vi "main.vi"() -> ()   [LabVIEW 2009]
uses:
  subvi/activity_info.vi
  <vilib>/Utility/file.llb/Write To Spreadsheet File (DBL).vi
  <vilib>/Utility/sysdir.llb/System Directory Type.ctl
panel:
  out "Primary and secondary axis power":dbl[](array[slide]) scale=0.0..800.0
  in  "Save Reference Signal to file":bool
  in  "Analysis Interval (s)":dbl(slide)=1.0 scale=0.0..4.0
  in  "Do ANN analysis":bool
  in  "Analysis Upperbound (minutes)":dbl(slide)=1000.0 scale=0.0..30.0
  out "minutes left":dbl
  out "minutes of execution":dbl
  out "case 3":i32
  out "case 2":i32
  out "case 1":i32
  out "case 0":i32
  out "output 2":dbl[](array[slide]) scale=0.0..1.0
  out "Correlations":cluster{dbl[], "correlation array":dbl[]}(graph)
  in  "Slide":cluster{dbl, dbl}(slide)={0.0, 1.0} scale=0.0..1.0
  out "above threshold":dbl(slide) scale=0.0..1.0
  in  "Threshold":dbl(slide)=0.85 scale=0.0..1.0
  out "Analyzing":u8(slide) scale=0.0..100.0
  in  "analyze correlations":bool
  in  "Reference Signal":i32
  in  "Reference Signals":dbl[][](array[numeric])
  in  "Save as reference Signal":bool
  in  "read weights":bool
  in  "Path":path=path "E:/Sensor/data/Phase II Data/csv format/Ara/Ara Walking.csv"
  out "C":bool
  out "B":bool
  out "A":bool
  in  "write data":bool
  out "Fundamental frequency":dbl(slide) scale=0.0..6.0
  in  "Normalize":bool
  in  "write to memory":bool
  out "activity output":u16(ring) items=["A", "B", "C", "D"]
  out "output":dbl[](array[slide]) scale=0.0..1.0
  in  "stop learning":bool
  out "Error (training)":dbl(graph)
  in  "Learning Rate":dbl(slide)=0.336734693877551 scale=0.0..1.0
  in  "Beta":dbl(slide)=1.0 scale=0.0..1.0
  in  "train":bool
  in  "Number of hidden neurons":i32(slide)=9 scale=0.0..20.0
  in  "delete state":bool
  in  "state":u32
  in  "activity":u16(ring) items=["A", "B", "C", "D", "E", "F", "G", "H"]
  in  "save state":bool
  in  "Tab Control":T1(tab)=enum."FFT on data 1"
  out "Time data on X',Y',Z'":T2(graph)
  out "FFT on X',Y',Z'":T3(graph)
  out "Filtered signal":dbl[](graph)
  out "Magnitude of time data":cluster{dbl[], dbl[]}(graph)
  out "activity states":T4(graph)
  in  "Sensor":u16(ring)=1 items=["Sensor 1", "Sensor 2", "Sensor 3"]
  in  "Sensor Type":u16(ring) items=["Acceleration", "Rotation"]
  in  "Sensor Brand":u16(ring)=1 items=["ADXL", "Kinetisense"]
  in  "End time (s) 1":dbl(slide)=10.0 scale=0.0..600.0
  in  "FFT interval (s) 1":dbl(slide)=4.0 scale=0.0..40.0
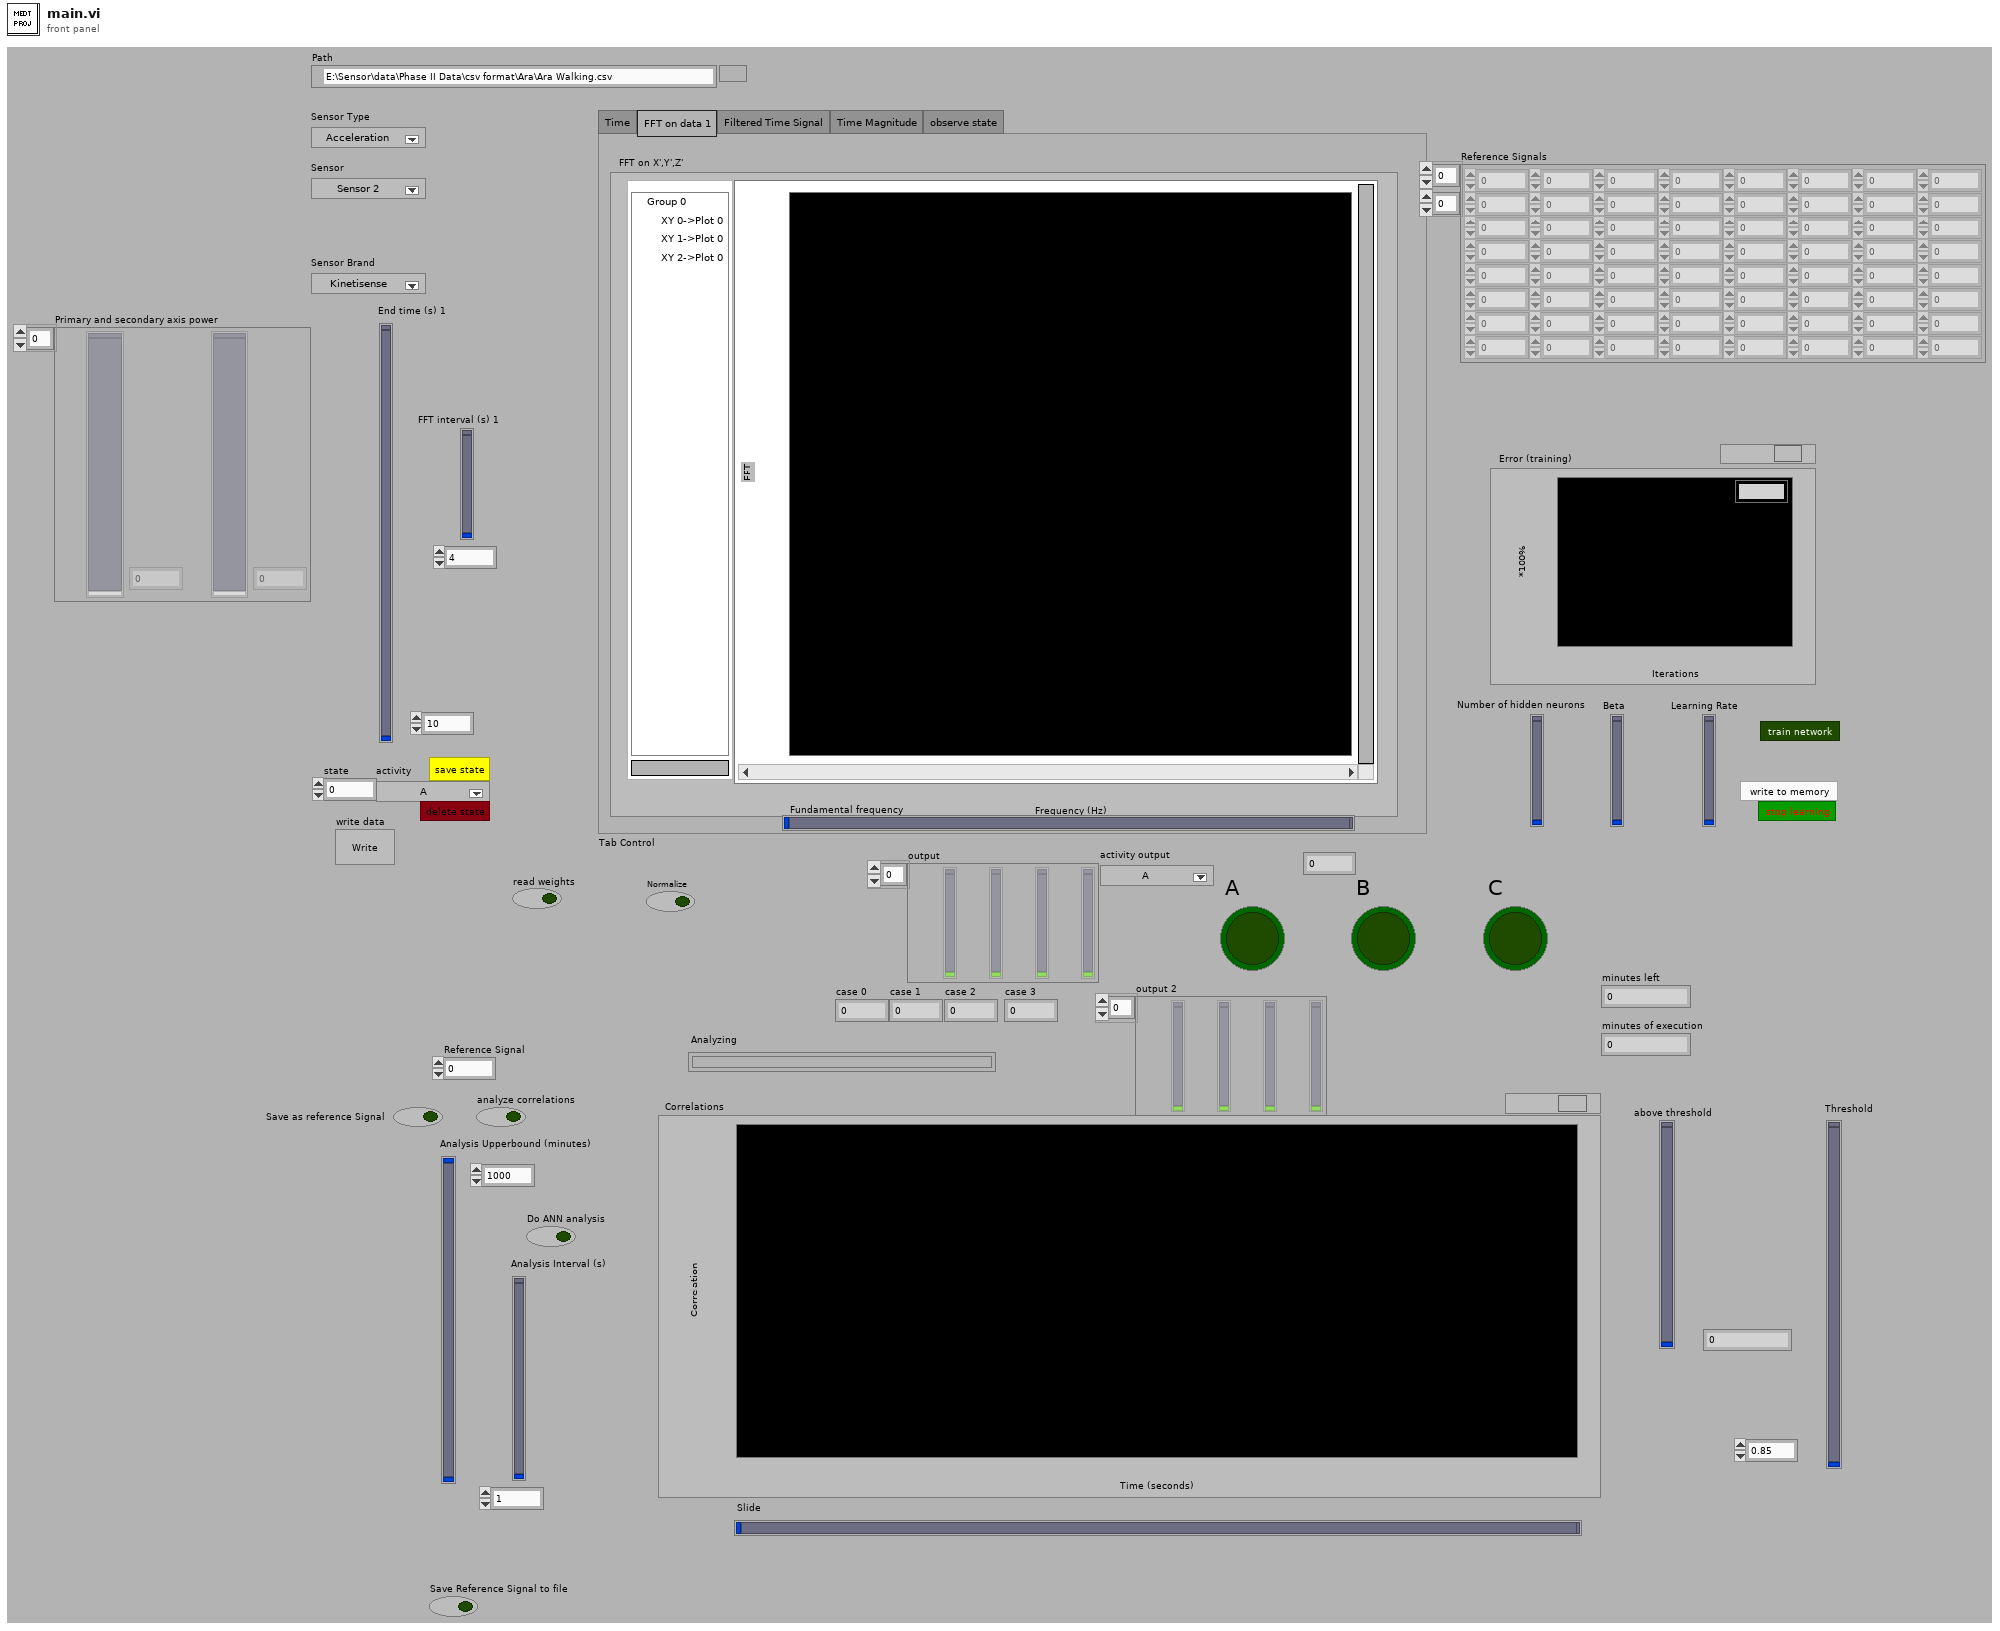
[diagram p1: front panel]
types:
  T1 = enum32{"Time", "FFT on data 1", "Filtered Time Signal", "Time Magnitude", "observe state"}
  T2 = cluster{cluster{dbl[], "Data out":dbl[]}, cluster{dbl[], "Data out":dbl[]}, cluster{dbl[], "Data out":dbl[]}}
  T3 = cluster{"XY Graph":cluster{dbl[], "magnitude":dbl[]}, "XY Graph":cluster{dbl[], "magnitude":dbl[]}, "XY Graph":cluster{dbl[], "magnitude":dbl[]}}
  T4 = cluster{cluster{dbl[], "Bicycling":dbl[]}, cluster{dbl[], "Bicycling":dbl[]}, cluster{dbl[], dbl[]}, cluster{dbl[], dbl[]}, cluster{dbl[], dbl[]}}
  T5 = typedef "System Directory Type.ctl" = i32
  T6 = cluster{"correlation array":dbl[], "correlation array":dbl[]}
  T7 = cluster{"A":dbl[][], "B":dbl[][], "C":dbl[][], "D":dbl[][]}
  T8 = cluster{cluster{dbl[], dbl[]}, cluster{dbl[], dbl[]}, cluster{dbl[], dbl[]}}
  T9 = cluster{"Cluster":cluster{dbl[], "activity":dbl[]}, "Cluster":cluster{dbl[], "activity":dbl[]}, cluster{dbl[], dbl[]}, cluster{dbl[], dbl[]}, cluster{dbl[], dbl[]}}
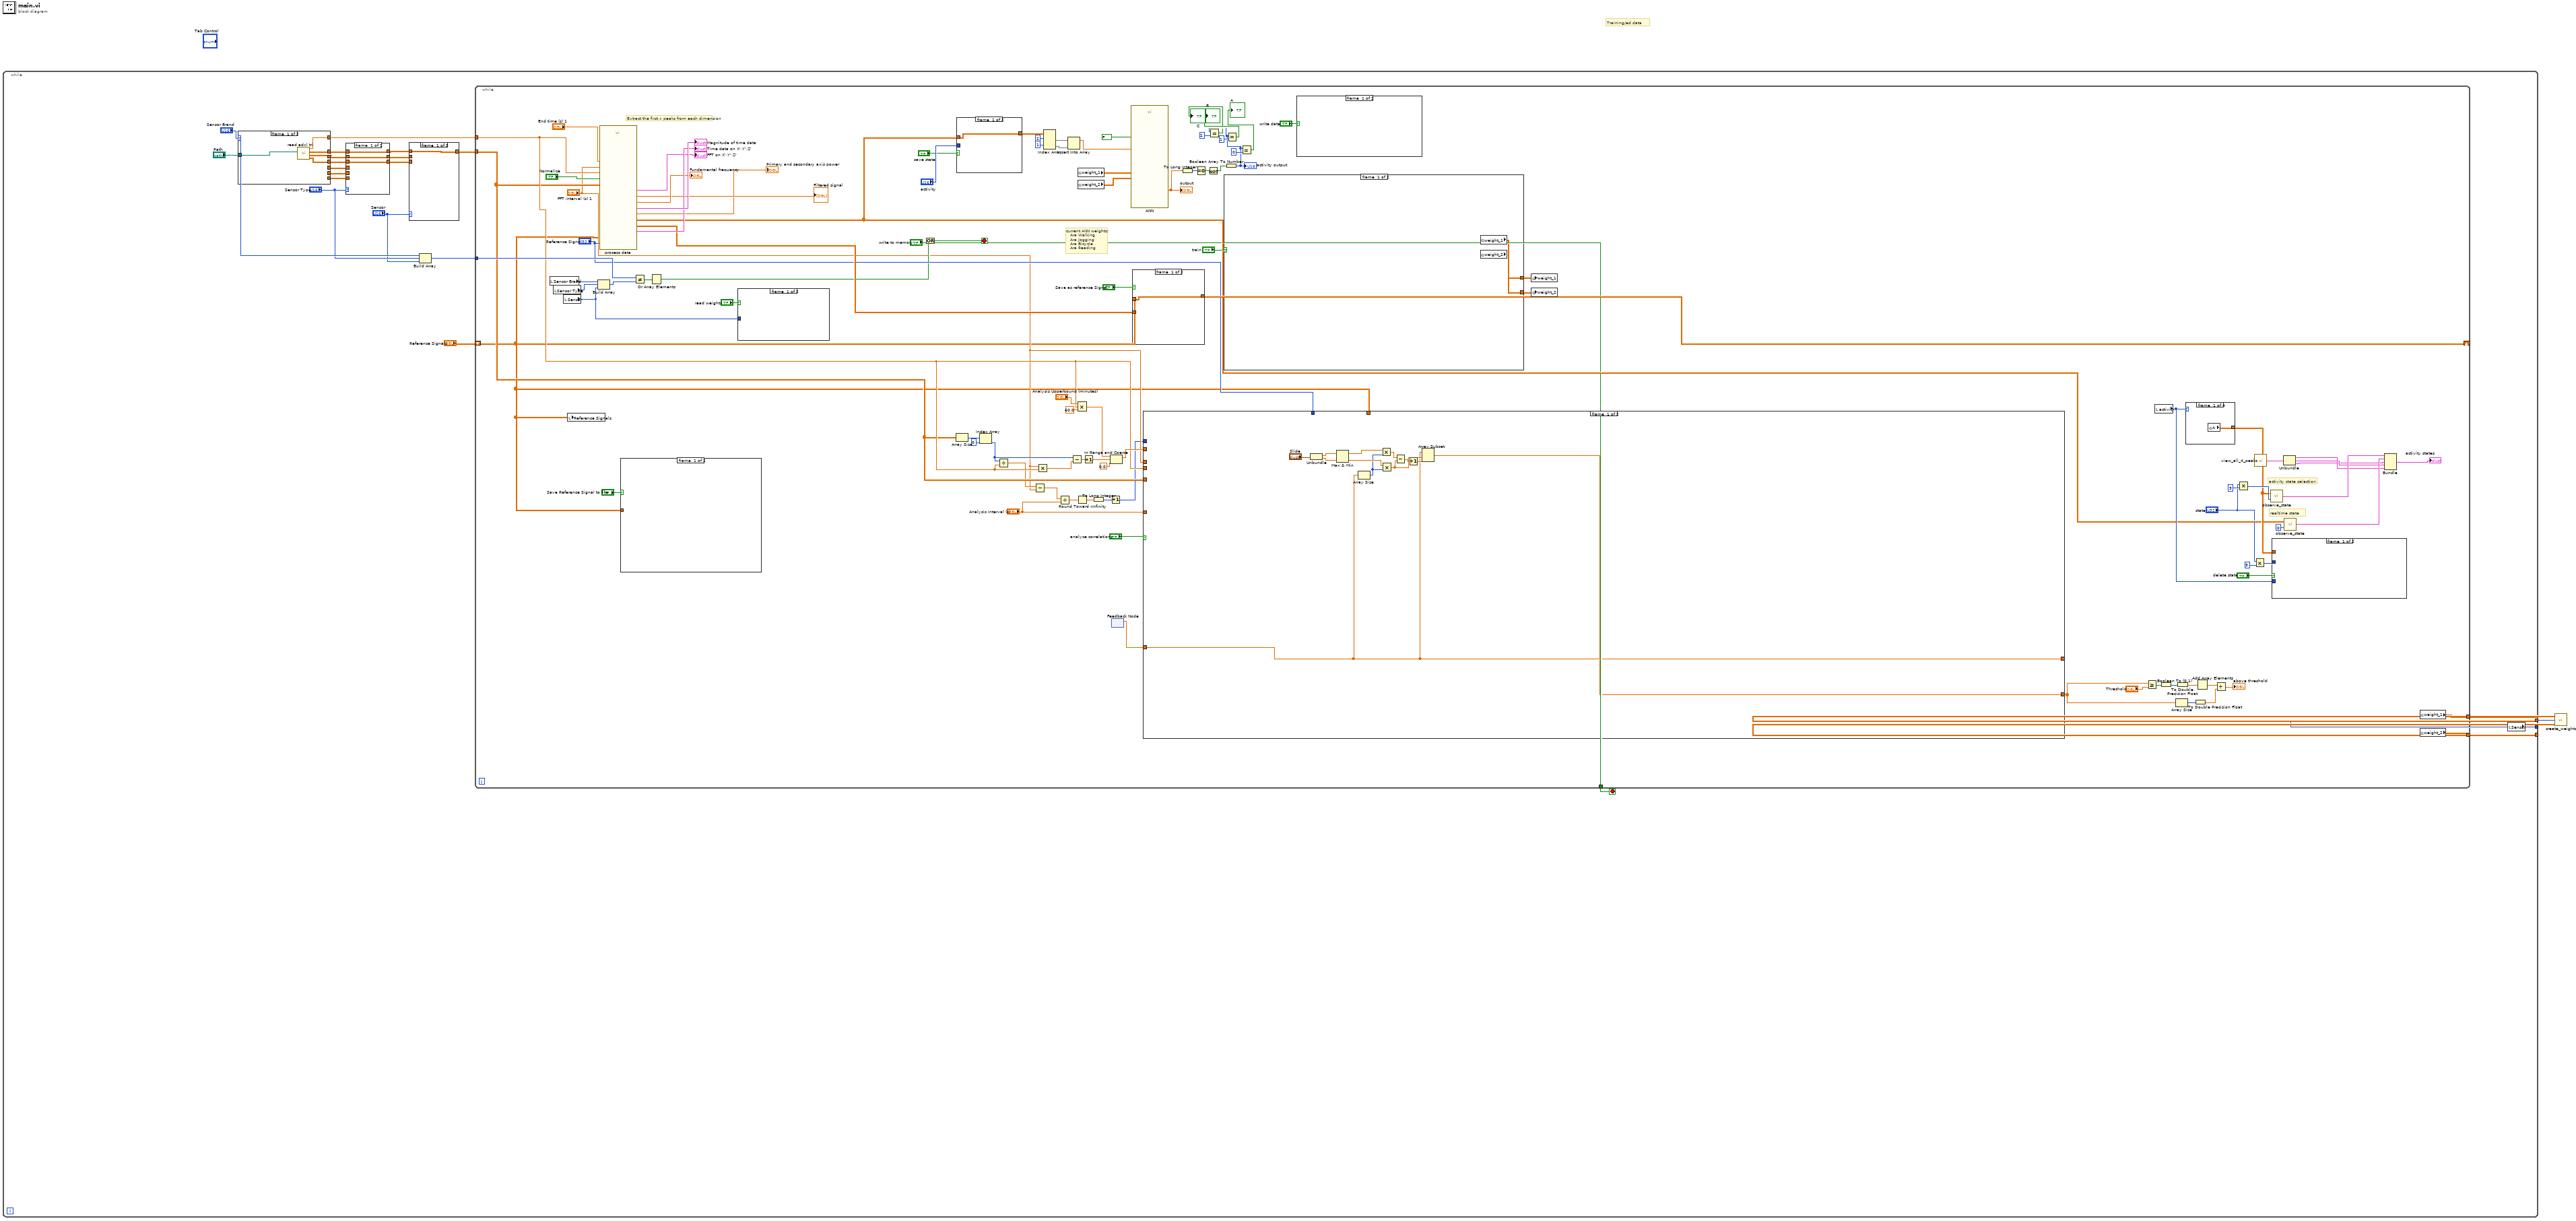
[diagram p0: block diagram]
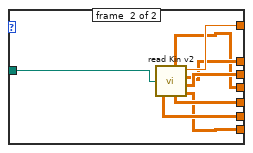
[diagram p5: hidden frame]
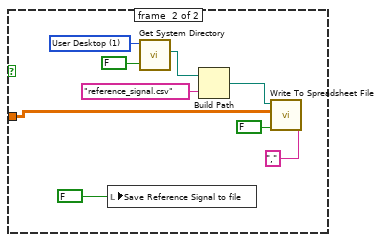
[diagram p6: hidden frame]
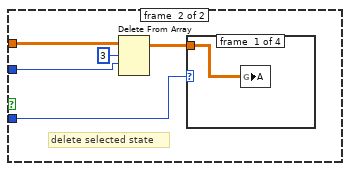
[diagram p7: hidden frame]
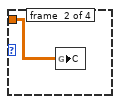
[diagram p8: hidden frame]
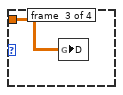
[diagram p9: hidden frame]
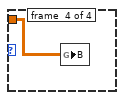
[diagram p10: hidden frame]
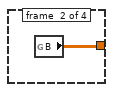
[diagram p11: hidden frame]
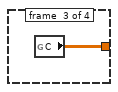
[diagram p12: hidden frame]
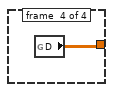
[diagram p13: hidden frame]
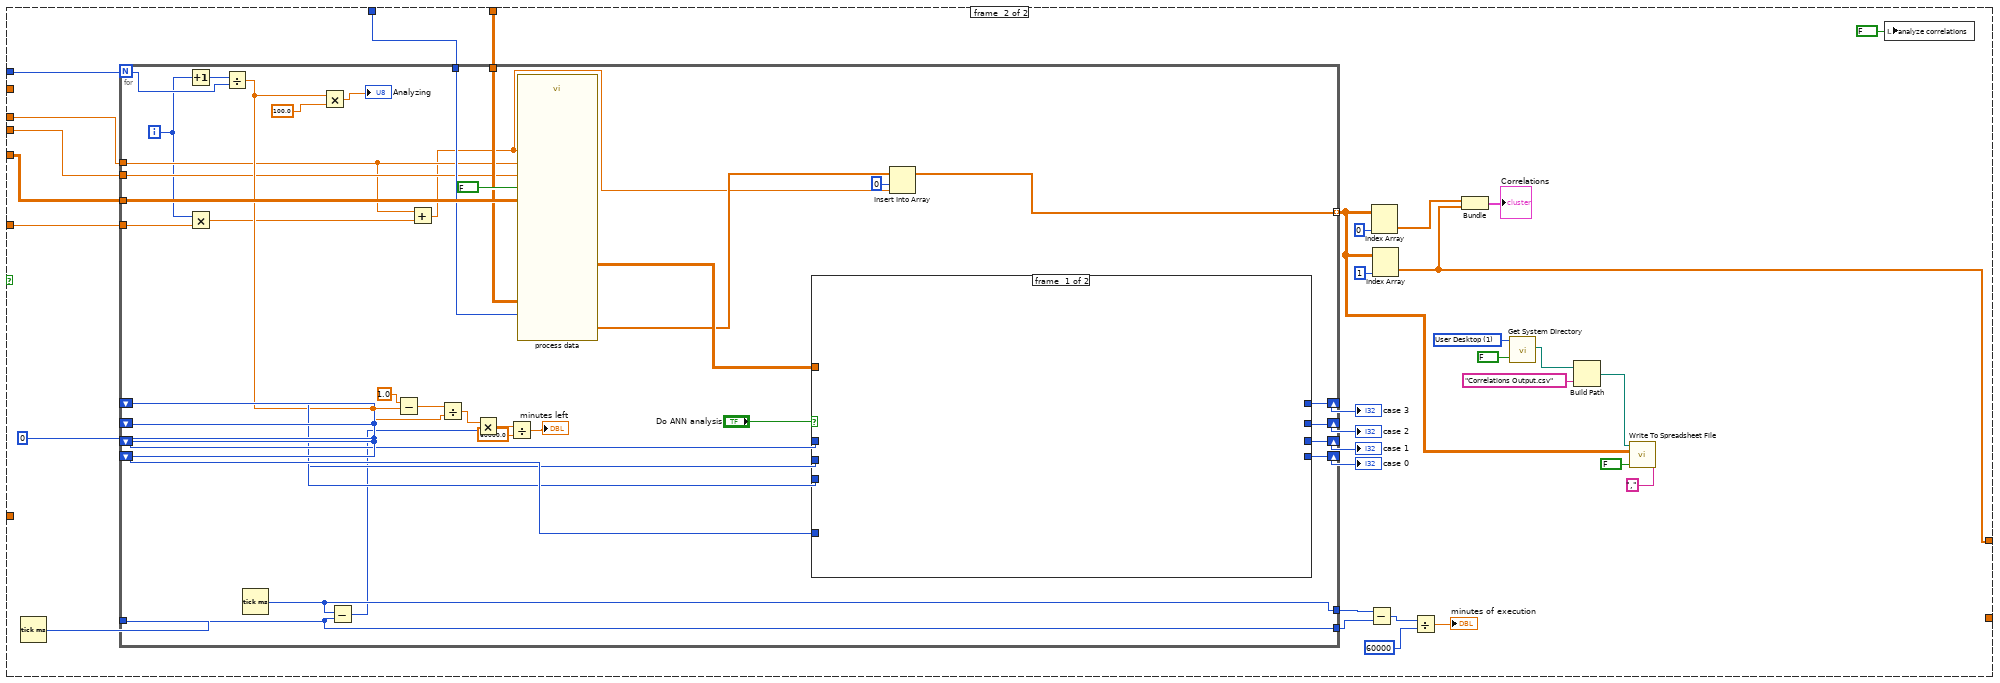
[diagram p14: hidden frame]
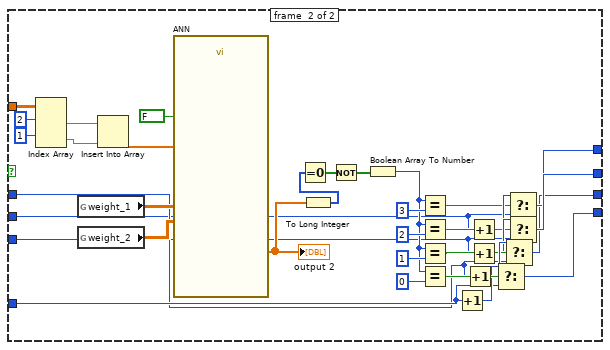
[diagram p15: hidden frame]
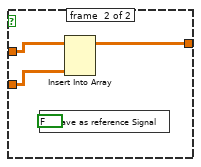
[diagram p16: hidden frame]
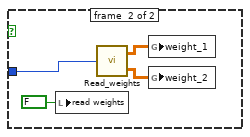
[diagram p17: hidden frame]
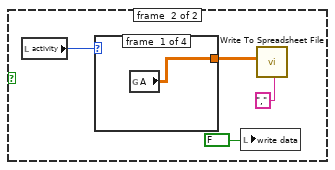
[diagram p18: hidden frame]
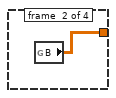
[diagram p19: hidden frame]
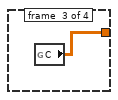
[diagram p20: hidden frame]
diagram:
  # "Training/ed data"
  n1 = while {
    tunnel: [w5] -> w3
    tunnel: [w4] -> w2
    tunnel: [w20] -> w1
    stop <- w21 stop-if-true
    n2 = case shown="1" "Sensor Brand" {
      tunnel: [w38 w46] -> w24
      tunnel: [w37 w45] -> w18
      tunnel: [w36 w44] -> w19
      tunnel: [w35 w43] -> w17
      tunnel: [_ w42] -> w16
      tunnel: [_ w41] -> w15
      tunnel: [_ w40] -> w14
      tunnel: "Path" -> [w34 w39]
      frame #0 {
        n3 = call "read adxl tri.vi"("file path"=w34) -> ("sensor 3 acceleration"=w35:dbl[][], "sensor 2 acceleration"=w37:dbl[][], "sensor 1 acceleration"=w36:dbl[][], "Frequency (Hz)"=w38:dbl)  [unwired: 4 in]
      }
      frame #1 {
        n4 = call "read Kin v2.vi"("file path"=w39) -> ("sensor 3 rotation"=w40:dbl[][], "sensor 1 rotation"=w42:dbl[][], "sensor 2 acceleration"=w45:dbl[][], "sensor 1 acceleration"=w44:dbl[][], "sensor 3 acceleration"=w43:dbl[][], "Frequency (Hz)"=w46:dbl, "sensor 2 rotation"=w41:dbl[][])  [unwired: 1 in]
      }
    }
    n5 = case shown="0, Default" "Sensor Type" {
      tunnel: w19 -> [w30 _]
      tunnel: w18 -> [w29 _]
      tunnel: w17 -> [w28 _]
      tunnel: w16 -> [_ w33]
      tunnel: w15 -> [_ w32]
      tunnel: w14 -> [_ w31]
      tunnel: [w30 w33] -> w8
      tunnel: [w29 w32] -> w13
      tunnel: [w28 w31] -> w12
      frame #0 {
      }
      frame #1 {
      }
    }
    n6 = case shown="1" "Sensor" {
      tunnel: w8 -> [w25 _ _]
      tunnel: w13 -> [_ w26 _]
      tunnel: w12 -> [_ _ w27]
      tunnel: [w25 w26 w27] -> w23
      frame #0 {
      }
      frame #1 {
      }
      frame #2 {
      }
    }
    n7 = Build Array("Sensor Brand", "Sensor Type", "Sensor") -> (w22:u16[])
    n8 = while {
      tunnel: w24 -> [w56]
      tunnel: w23 -> [w55]
      tunnel: w22 -> [w140]
      tunnel: ["write to memory"] -> w21
      shift-right: [w106] -> _
      shift-left: "Reference Signals" -> [w48]
      tunnel: [w70] -> w5
      tunnel: [w69] -> w4
      stop <- w121 stop-if-true
      # "activity state selection"
      # "realtime state"
      # "current ANN weights:\n   Ara Walking\n   Ara Jogging\n   Ara Bicycle\n   Ara Reading"
      # "Extract the first x peaks from each dimension"
      n9 = local read "Sensor Brand"() -> (w144:u16)
      n10 = local read "Sensor Type"() -> (w143:u16)
      n11 = local read "Sensor"() -> (w109:u16)
      n12 = local write "Reference Signals"(w48) -> ()
      n13 = Build Array(w144, w143, w109) -> (w142:u16[])
      n14 = call "process data.vi"("Frequency (Hz)"=w56, "Reference Signal"="Reference Signal", "sensor input"=w55, "In Signals"=w48, "FFT interval (s)"="FFT interval (s) 1", "Normalize"="Normalize", "End time (s)"="End time (s) 1") -> ("Fundamental frequency"=→"Fundamental frequency":dbl, "FFT"=→"FFT on X',Y',Z'":T3, "peaks"=w74:dbl[][], "Magnitude of time data"=→"Magnitude of time data":cluster{dbl[], dbl[]}, "x',y',z'"=→"Time data on X',Y',Z'":T2, "Signals"=w105:dbl[][], "Filtered signal"=→"Filtered signal":dbl[], "Primary and secondary axis power"=→"Primary and secondary axis power":dbl[])  [unwired: 1 out]
      n15 = case shown="True" "Save Reference Signal to file" {
        tunnel: w48 -> [_ w152]
        frame #0 {
        }
        frame #1 {
          w157 = T5 1 items=["User Home", "User Desktop", "User Documents", "User Application Data", "User Preferences", "User Temporary", "Public Documents", "Public Application Data", "Public Preferences", "System Core Libraries", "System Installed Libraries", "Application Files", "Boot Volume Root"] ("system directory type")
          n16 = local write "Save Reference Signal to file"(FALSE ("Save Reference Signal")) -> ()
          n17 = call <vilib>:"Get System Directory.vi"("create directory if not found? (F)"=FALSE, "system directory type"=w157) -> ("system directory"=w154:path)  [unwired: 9 in]
          n18 = Build Path(base path=w154, name or relative path="reference_signal.csv") -> (appended path=w153:path)
          n19 = call-poly <vilib>:"Write To Spreadsheet File.vi"("delimiter (\\t)"="," ("delimiter (\\t)"), "append to file? (new file:F)"=FALSE, "2D data"=w152, "file path (dialog if empty)"=w153) -> ()  [unwired: 4 in, 1 out]
        }
      }
      n20 = Not Equal?(x=w140, y=w142) -> (x != y?=w141:bool[])
      n21 = Or Array Elements(Boolean array=w141) -> (logical OR=w75:bool)
      n22 = case shown="True" "read weights" {
        tunnel: w109 -> [_ w294]
        frame #0 {
        }
        frame #1 {
          n23 = local write "read weights"(FALSE ("read weights")) -> ()
          n24 = call "Read_weights.vi"("sensor"=w294) -> ("weights 1"=w292:dbl[][], "weights 2"=w291:dbl[][])
          n25 = global write "activity_info.vi" "weight_1"(w292) -> ()
          n26 = global write "activity_info.vi" "weight_2"(w291) -> ()
        }
      }
      n27 = Or(x=w75, y="write to memory") -> (x .or. y?=w121:bool)
      n28 = Array Size(array=w55) -> (size(s)=w104:i32[])
      n29 = case shown="True" "save state" {
        tunnel: w74 -> [w326 w328]
        tunnel: [w326 w328] -> w131
        tunnel: "activity" -> [_ w327]
        frame #0 {
        }
        frame #1 {
          # "save the state to  temp memory"
          n30 = call "save_state.vi"("state"=w327, "peaks"=w328) -> ()  [unwired: 1 in]
        }
      }
      n31 = Index Array(array=w104, index=0) -> (element=w60:i32)
      n32 = Divide(x=w60, y=w56) -> (x/y=w54:dbl)
      n33 = Subtract(x=w54, y="FFT interval (s) 1") -> (x-y=w52:dbl)
      n34 = Multiply(x="FFT interval (s) 1", y=w56) -> (x*y=w102:dbl)
      n35 = Index Array(array=w131, index (row) #1=2 ("index (row)"), index (row) #2=1 ("index (row)")) -> (element #1=w134:dbl[], element #2=w133:dbl[])  [unwired: 2 in]
      n36 = Divide(x=w52, y="Analysis Interval (s)") -> (x/y=w59:dbl)
      n37 = Insert Into Array(array=w134, new element=w133) -> (w132:dbl[])  [unwired: 1 in]
      n38 = Subtract(x=w60, y=w102) -> (x-y=w101:dbl)
      n39 = Round Toward -Infinity(1:w59) -> (0:w58:dbl)
      n40 = global read "activity_info.vi" "weight_1"() -> (w130:dbl[][])
      n41 = global read "activity_info.vi" "weight_2"() -> (w129:dbl[][])
      n42 = Compound Arithmetic op=MULTIPLY("Analysis Upperbound (minutes)", w56, 60.0 ("value")) -> (w63:dbl)
      n43 = Increment(x=w101) -> (x+1=w65:dbl)
      n44 = To Long Integer(number=w58) -> (32bit integer=w51:i32)
      n45 = Increment(x=w51) -> (x+1=w50:i32)
      n46 = In Range and Coerce(upper limit=w63, x=w65, lower limit=0.0) -> (coerced(x)=w62:dbl)  [unwired: 1 out]
      n47 = feedback #1() -> (w89:dbl[])  [unwired: 1 in]
      n48 = call "ANN.vi"("Input"=w132, "Weight_2"=w129, "Weight_1"=w130, "Back Propagation"=FALSE) -> ("output"=w125:dbl[])  [unwired: 8 in, 3 out]
      "output" <- w125
      n49 = case shown="True" "Save as reference Signal" {
        tunnel: w105 -> [_ w290]
        tunnel: [w286 w287] -> w106
        tunnel: w48 -> [w286 w288]
        frame #0 {
        }
        frame #1 {
          n50 = local write "Save as reference Signal"(FALSE ("Save Signal")) -> ()
          n51 = Insert Into Array(array=w288, new element=w290) -> (w287:dbl[][])  [unwired: 2 in]
        }
      }
      n52 = case shown="True" "analyze correlations" {
        tunnel: w55 -> [_ w214]
        tunnel: w56 -> [_ w209]
        tunnel: "FFT interval (s) 1" -> [_ w187]
        tunnel: w62 -> [_ _]
        tunnel: w48 -> [_ w213]
        tunnel: "Reference Signal" -> [_ w210]
        tunnel: [w172 w183] -> w90
        tunnel: w89 -> [w172 _]
        tunnel: [w171 _] -> w61
        tunnel: w50 -> [_ w189]
        tunnel: "Analysis Interval (s)" -> [_ w188]
        frame #0 {
          n53 = Unbundle("Slide") -> (w181:dbl, w180:dbl)
          n54 = Max & Min(x=w181, y=w180) -> (max(x,y)=w177:dbl, min(x,y)=w179:dbl)
          n55 = Array Size(array=w172) -> (size(s)=w178:i32)
          n56 = Multiply(x=w177, y=w178) -> (x*y=w176:dbl)
          n57 = Multiply(x=w179, y=w178) -> (x*y=w175:dbl)
          n58 = Subtract(x=w176, y=w175) -> (x-y=w173:dbl)
          n59 = Increment(x=w173) -> (x+1=w174:dbl)
          n60 = Array Subset(array=w172, index=w175, length=w174) -> (w171:dbl[])
        }
        frame #1 {
          w194 = T5 1 items=["User Home", "User Desktop", "User Documents", "User Application Data", "User Preferences", "User Temporary", "Public Documents", "Public Application Data", "Public Preferences", "System Core Libraries", "System Installed Libraries", "Application Files", "Boot Volume Root"] ("system directory type")
          w207 = 0
          n61 = Tick Count (ms)() -> (millisecond timer value=w202:u32)
          n62 = for {
            N: w189 -> [w248]
            tunnel: w214 -> [w250]
            tunnel: w187 -> [w221]
            tunnel: w209 -> [w223]
            tunnel: [w215] -> w185 mode=indexing
            tunnel: w213 -> [w249]
            tunnel: w210 -> [w245]
            shift-right: [w242] -> w206
            shift-left: w207 -> [w243]
            shift-right: [w236] -> w205
            shift-left: w207 -> [w241]
            shift-right: [w239] -> w204
            shift-left: w207 -> [w240]
            shift-right: [w237] -> w203
            shift-left: w207 -> [w238]
            tunnel: w202 -> [w234]
            tunnel: [w234] -> w201
            tunnel: [w235] -> w197
            tunnel: w188 -> [w224]
            i -> [w220]
            n63 = Increment(x=w220) -> (x+1=w219:i32)
            n64 = Multiply(x=w220, y=w224) -> (x*y=w222:dbl)
            n65 = Divide(x=w219, y=w248) -> (x/y=w231:dbl)
            n66 = Tick Count (ms)() -> (millisecond timer value=w235:u32)
            n67 = Multiply(x=w231, y=100.0) -> (x*y=→"Analyzing":dbl)
            n68 = Subtract(x=w235, y=w234) -> (x-y=w229:u32)
            n69 = Subtract(x=1.0, y=w231) -> (x-y=w232:dbl)
            n70 = Add(x=w221, y=w222) -> (x+y=w217:dbl)
            n71 = Divide(x=w232, y=w231) -> (x/y=w230:dbl)
            n72 = Multiply(x=w230, y=w229) -> (x*y=w228:dbl)
            n73 = Divide(x=w228, y=60000.0) -> (x/y=→"minutes left":dbl)
            n74 = call "process data.vi"("Frequency (Hz)"=w223, "Reference Signal"=w245, "sensor input"=w250, "In Signals"=w249, "FFT interval (s)"=w221, "Normalize"=FALSE, "End time (s)"=w217) -> ("peaks"=w244:dbl[][], "correlation array"=w218:dbl[])  [unwired: 7 out]
            n75 = case shown="False" "Do ANN analysis" {
              tunnel: w244 -> [_ w276]
              tunnel: w243 -> [_ w265]
              tunnel: [_ w264] -> w242
              tunnel: w241 -> [_ w261]
              tunnel: w240 -> [_ w258]
              tunnel: [_ w257] -> w239
              tunnel: w238 -> [_ w254]
              tunnel: [_ w253] -> w237
              tunnel: [_ w252] -> w236
              frame #0 {
              }
              frame #1 {
                n76 = Index Array(array=w276, index (row) #1=2 ("index (row)"), index (row) #2=1 ("index (row)")) -> (element #1=w282:dbl[], element #2=w281:dbl[])  [unwired: 2 in]
                n77 = global read "activity_info.vi" "weight_1"() -> (w279:dbl[][])
                n78 = global read "activity_info.vi" "weight_2"() -> (w278:dbl[][])
                n79 = Insert Into Array(array=w282, new element=w281) -> (w280:dbl[])  [unwired: 1 in]
                n80 = call "ANN.vi"("Input"=w280, "Weight_2"=w278, "Weight_1"=w279, "Back Propagation"=FALSE) -> ("output"=w277:dbl[])  [unwired: 8 in, 3 out]
                "output 2" <- w277
                n81 = To Long Integer(number=w277) -> (32bit integer=w274:i32[])
                n82 = Equal To 0?(x=w274) -> (x = 0?=w275:bool[])
                n83 = Not(x=w275) -> (.not. x?=w273:bool[])
                n84 = Boolean Array To Number(Boolean array=w273) -> (number=w268:u32)
                n85 = Equal?(x=w268, y=3) -> (x = y?=w255:bool)
                n86 = Equal?(x=w268, y=2) -> (x = y?=w259:bool)
                n87 = Equal?(x=w268, y=1) -> (x = y?=w262:bool)
                n88 = Equal?(x=w268, y=0) -> (x = y?=w267:bool)
                n89 = Increment(x=w265) -> (x+1=w266:i32)
                n90 = Increment(x=w261) -> (x+1=w263:i32)
                n91 = Increment(x=w254) -> (x+1=w256:i32)
                n92 = Increment(x=w258) -> (x+1=w260:i32)
                n93 = Select(t=w266, s=w267, f=w265) -> (s? t:f=w264:i32)
                n94 = Select(t=w263, s=w262, f=w261) -> (s? t:f=w252:i32)
                n95 = Select(t=w256, s=w255, f=w254) -> (s? t:f=w253:i32)
                n96 = Select(t=w260, s=w259, f=w258) -> (s? t:f=w257:i32)
              }
            }
            n97 = Insert Into Array(array=w218, index=0, new element=w217) -> (w215:dbl[])
          }
          "case 0" <- w206
          "case 1" <- w205
          "case 2" <- w204
          "case 3" <- w203
          n98 = Subtract(x=w197, y=w201) -> (x-y=w200:u32)
          n99 = Index Array(array=w185, index (col)=0 ("disabled index (col)")) -> (element=w184:dbl[])  [unwired: 1 in]
          n100 = Index Array(array=w185, index (col)=1 ("disabled index (col)")) -> (element=w183:dbl[])  [unwired: 1 in]
          n101 = Divide(x=w200, y=u32 60000) -> (x/y=→"minutes of execution":dbl)
          n102 = Bundle("correlation array"=w184, "correlation array"=w183) -> (→"Correlations":T6)  [unwired: 1 in]
          n103 = call <vilib>:"Get System Directory.vi"("create directory if not found? (F)"=FALSE, "system directory type"=w194) -> ("system directory"=w192:path)  [unwired: 9 in]
          n104 = Build Path(base path=w192, name or relative path="Correlations Output.csv") -> (appended path=w191:path)
          n105 = call-poly <vilib>:"Write To Spreadsheet File.vi"("delimiter (\\t)"="," ("delimiter (\\t)"), "append to file? (new file:F)"=FALSE, "2D data"=w185, "file path (dialog if empty)"=w191) -> ()  [unwired: 4 in, 1 out]
          n106 = local write "analyze correlations"(FALSE ("analyze correlations")) -> ()
        }
      }
      n107 = To Long Integer(number=w125) -> (32bit integer=w124:i32[])
      n108 = Equal To 0?(x=w124) -> (x = 0?=w123:bool[])
      n109 = Not(x=w123) -> (.not. x?=w122:bool[])
      n110 = case shown="True" "train" {
        tunnel: [w303 w308] -> w128
        tunnel: [w304 w307] -> w127
        frame #0 {
          n111 = global read "activity_info.vi" "weight_1"() -> (w304:dbl[][])
          n112 = global read "activity_info.vi" "weight_2"() -> (w303:dbl[][])
        }
        frame #1 {
          # "# of inputs +1"
          # "# of outputs"
          n113 = call "initial weights.vi"("Number of classifiers"=3, "Number of hidden neurons"="Number of hidden neurons", "Inputs + 1"=9) -> ("Weights 2"=w316:dbl[][], "Weights 1"=w315:dbl[][])
          n114 = global read "activity_info.vi" "D"() -> (w309:dbl[][])
          n115 = global read "activity_info.vi" "C"() -> (w313:dbl[][])
          n116 = global read "activity_info.vi" "B"() -> (w312:dbl[][])
          n117 = global read "activity_info.vi" "A"() -> (w306:dbl[][])
          n118 = Bundle("A"=w306, "B"=w312, "C"=w313, "D"=w309) -> (w314:T7)  [unwired: 1 in]
          n119 = while {
            tunnel: w314 -> [w317]
            shift-right: [w323] -> w307
            shift-left: w315 -> [w325]
            shift-right: [w322] -> w308
            shift-left: w316 -> [w324]
            stop <- "stop learning" stop-if-true
            n120 = call "learning_phase.vi"("Weights 2"=w324, "Weights 1"=w325, "Learning Rate"="Learning Rate", "Beta"="Beta", "inputs"=w317) -> ("Error"=→"Error (training)":dbl, "Weight_2_out"=w322:dbl[][], "Weight_1_out"=w323:dbl[][])
          }
        }
      }
      n121 = Boolean Array To Number(Boolean array=w122) -> (number=w113:u32)
      "activity output" <- w113
      n122 = Equal?(x=w113, y=u32 2) -> (x = y?=→"C":bool)
      n123 = Equal?(x=w113, y=u32 1) -> (x = y?=→"B":bool)
      n124 = Equal?(x=w113, y=u32 0) -> (x = y?=→"A":bool)
      n125 = case shown="True" "write data" {
        frame #0 {
        }
        frame #1 {
          n126 = local read "activity"() -> (w298:u16)
          n127 = case shown="0, Default" w298 {
            tunnel: [w299 w300 w301 w302] -> w297
            frame #0 {
              n128 = global read "activity_info.vi" "A"() -> (w299:dbl[][])
            }
            frame #1 {
              n129 = global read "activity_info.vi" "B"() -> (w300:dbl[][])
            }
            frame #2 {
              n130 = global read "activity_info.vi" "C"() -> (w301:dbl[][])
            }
            frame #3 {
              n131 = global read "activity_info.vi" "D"() -> (w302:dbl[][])
            }
          }
          n132 = local write "write data"(FALSE ("write data")) -> ()
          n133 = call-poly <vilib>:"Write To Spreadsheet File.vi"("delimiter (\\t)"="," ("delimiter (\\t)"), "2D data"=w297) -> ()  [unwired: 6 in, 1 out]
        }
      }
      n134 = global write "activity_info.vi" "weight_1"(w127) -> ()
      n135 = global write "activity_info.vi" "weight_2"(w128) -> ()
      n136 = Greater Or Equal?(x=w61, y="Threshold") -> (x >= y?=w92:bool[])
      n137 = local read "activity"() -> (w76:u16)
      n138 = Boolean To (0,1)(Boolean=w92) -> (0, 1=w93:i16[])
      n139 = Array Size(array=w61) -> (size(s)=w96:i32)
      n140 = To Double Precision Float(number=w93) -> (double precision float=w94:dbl[])
      n141 = case shown="3" w76 {
        tunnel: [w167 w168 w169 w170] -> w77
        frame #0 {
          n142 = global read "activity_info.vi" "A"() -> (w167:dbl[][])
        }
        frame #1 {
          n143 = global read "activity_info.vi" "B"() -> (w168:dbl[][])
        }
        frame #2 {
          n144 = global read "activity_info.vi" "C"() -> (w169:dbl[][])
        }
        frame #3 {
          n145 = global read "activity_info.vi" "D"() -> (w170:dbl[][])
        }
      }
      n146 = To Double Precision Float(number=w96) -> (double precision float=w97:dbl)
      n147 = Add Array Elements(numeric array=w94) -> (sum=w95:dbl)
      n148 = Divide(x=w95, y=w97) -> (x/y=→"above threshold":dbl)
      n149 = Multiply(x="state", y=u32 3) -> (x*y=w87:u32)
      n150 = Multiply(x="state", y=u32 3) -> (x*y=w84:u32)
      n151 = call "view_all_4_peaks.vi"("activity"=w77) -> ("Cluster"=w81:T8)
      n152 = call "observe_state.vi"("Numeric"=w87, "activity"=w77) -> ("Cluster"=w86:cluster{dbl[], "activity":dbl[]})
      n153 = case shown="True" "delete state" {
        tunnel: w77 -> [_ w162]
        tunnel: w84 -> [_ w160]
        tunnel: w76 -> [_ w159]
        frame #0 {
        }
        frame #1 {
          # "delete selected state"
          n154 = Delete From Array(array=w162, length=3, index (row)=w160) -> (array with subset deleted=w158:dbl[][])  [unwired: 1 in, 1 out]
          n155 = case shown="3" w159 {
            tunnel: w158 -> [w163 w164 w165 w166]
            frame #0 {
              n156 = global write "activity_info.vi" "A"(w163) -> ()
            }
            frame #1 {
              n157 = global write "activity_info.vi" "C"(w164) -> ()
            }
            frame #2 {
              n158 = global write "activity_info.vi" "D"(w165) -> ()
            }
            frame #3 {
              n159 = global write "activity_info.vi" "B"(w166) -> ()
            }
          }
        }
      }
      n160 = Unbundle(w81) -> (w80:cluster{dbl[], dbl[]}, w79:cluster{dbl[], dbl[]}, w78:cluster{dbl[], dbl[]})
      n161 = call "observe_state.vi"("Numeric"=u32 0, "activity"=w74) -> ("Cluster"=w82:cluster{dbl[], "activity":dbl[]})
      n162 = Bundle("Cluster"=w86, "Cluster"=w82, w78, w79, w80) -> (→"activity states":T9)  [unwired: 1 in]
      n163 = global read "activity_info.vi" "weight_1"() -> (w70:dbl[][])
      n164 = global read "activity_info.vi" "weight_2"() -> (w69:dbl[][])
    }
    n165 = local read "Sensor"() -> (w20:u16)
  }
  n166 = call "create_weights.vi"("weight2"=w2, "Ring"=w1, "weight1"=w3) -> ()
